vi "CompareTrial.vi"() -> ()   [LabVIEW 2012]
panel:
  out "DAC Output":dbl
  out "Input>Trial":bool
  in  "Trial Voltage":dbl
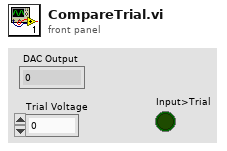
[diagram p1: front panel]
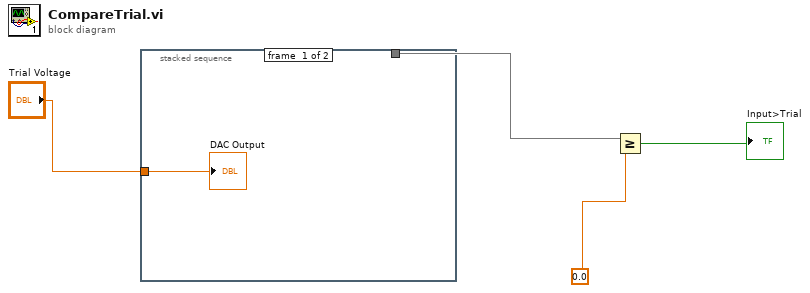
[diagram p0: block diagram]
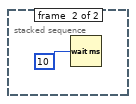
[diagram p2: hidden frame]
diagram:
  n1 = stacked-sequence {
    tunnel: "Trial Voltage" -> [w5 _]
    tunnel: [_ _] -> w2
    frame #0 {
      "DAC Output" <- w5
    }
    frame #1 {
      n2 = Wait (ms)(milliseconds to wait=10) -> ()  [unwired: 1 out]
    }
  }
  n3 = Greater Or Equal?(x=w2, y=0.0) -> (x >= y?=→"Input>Trial":bool)
